vi "SwerveHeadingLock.vi"(1 "Max Driver Translation Joystick":dbl, 3 "Driver Rotation Joystick":dbl, 6 "PID Tuning Parameters":T1={"Kp"=0.1, "Ki"=0.1, "Kd"=0.1, "N-Diff"=10, "N-Int"=20, "Int Error Window"=0.5, "Max Ouput"=1.0, "Min Output"=-1.0, "Square Derivative"=FALSE, "N-Prop"=1} {"N-Prop" min=1; "Int Error Window" min=0.0; "N-Int" min=2; "N-Diff" min=2; "Kd" min=0.0; "Ki" min=0.0; "Kp" min=0.0}, 8 "Deceleration Hysteresis (ms)":u32, 10 "Heading Lock Strafe Deadband (ft/s)":dbl, 12 "External Disables":bool) -> (14 "Controller Summary":T2(graph), 17 "Joystick Rotation":dbl, 19 "Heading Lock":bool)   [LabVIEW 2020]
doc: "This VI runs a PID controller to maintain the robot's heading while translating above a specified velocity. Dropping below the velocity threshold or manually commanding a rotation will switch off the heading lock. Assumes that all of the joystick deadbands and scalings have already been applied."
uses:
  sensordata.vi
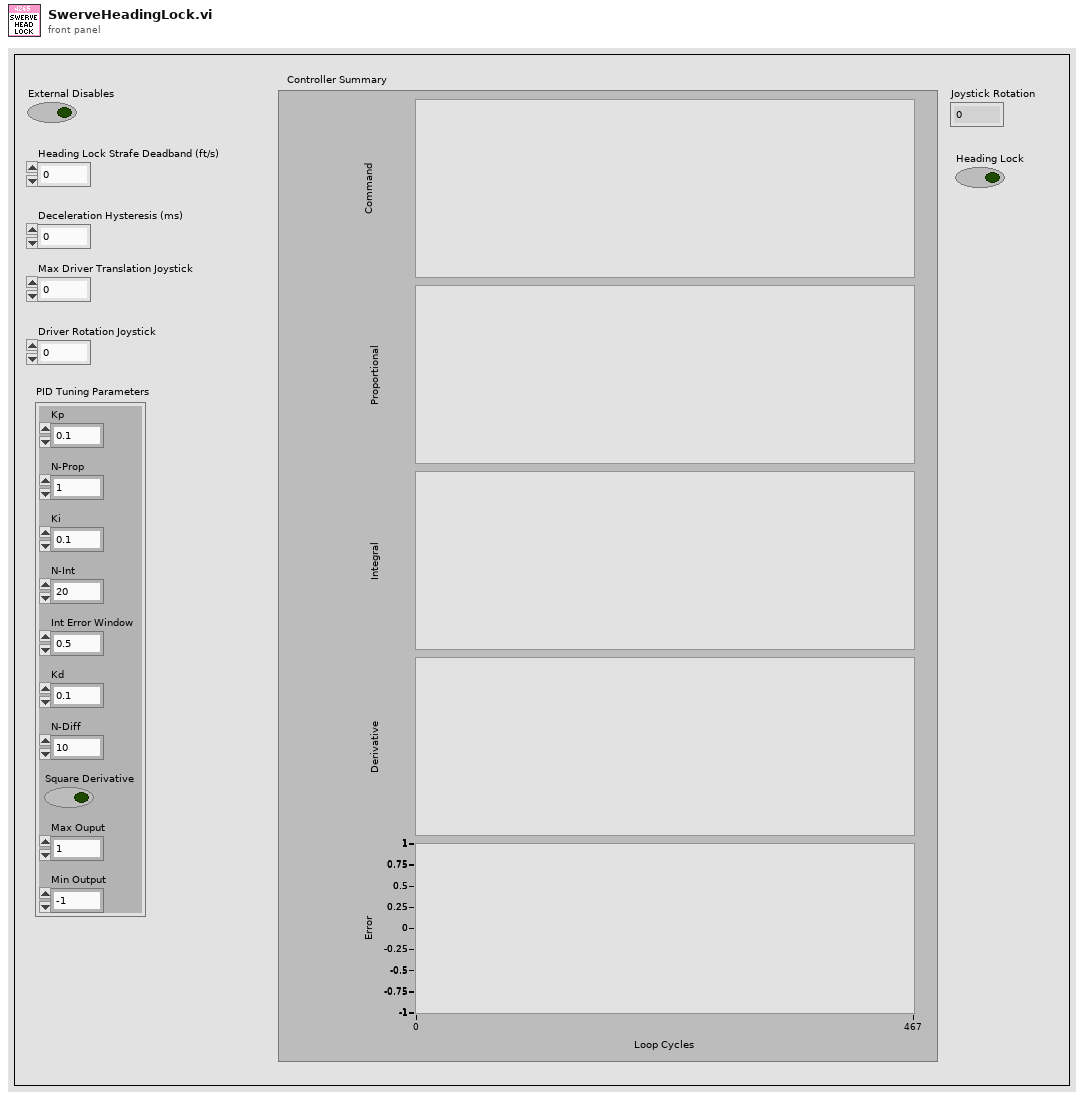
[diagram p1: front panel]
types:
  T1 = cluster{"Kp":dbl, "Ki":dbl, "Kd":dbl, "N-Diff":i32, "N-Int":i32, "Int Error Window":dbl, "Max Ouput":dbl, "Min Output":dbl, "Square Derivative":bool, "N-Prop":i32}
  T2 = cluster{"Command":dbl, "Proportional":dbl, "Integral":dbl, "Derivative":dbl, "Goal":dbl}
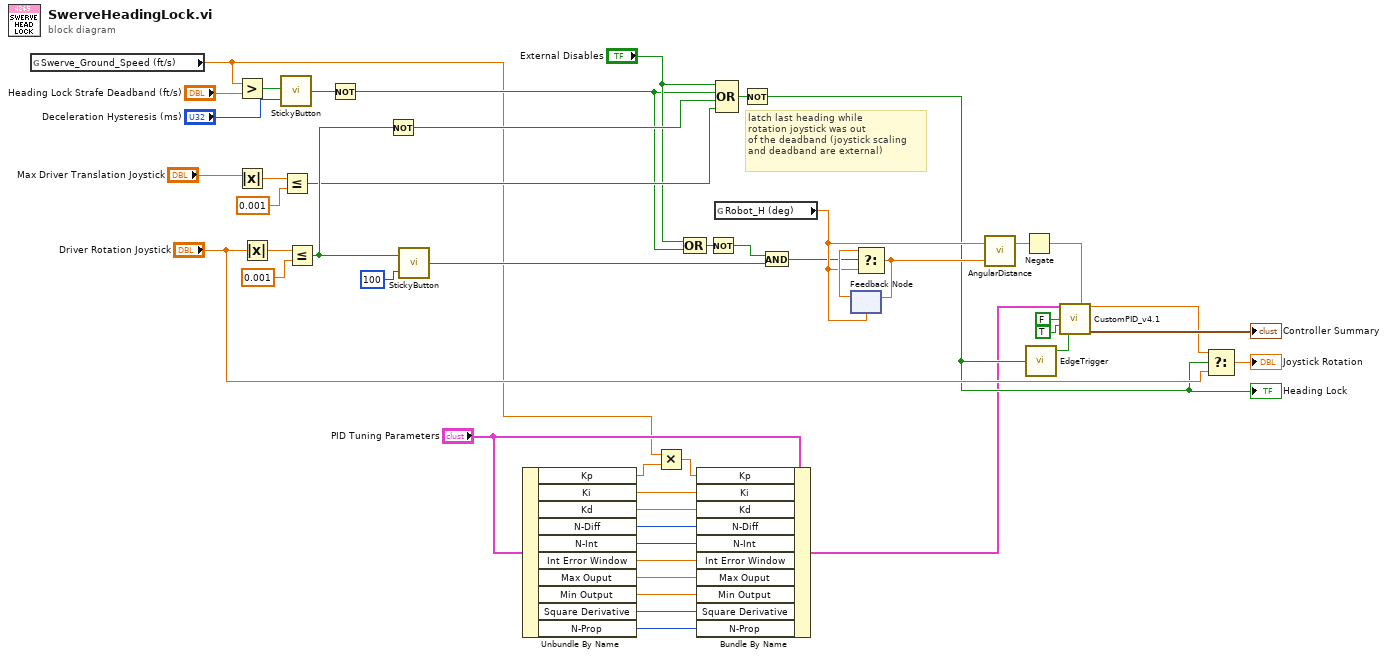
[diagram p0: block diagram]
diagram:
  # "latch last heading while\nrotation joystick was out \nof the deadband (joystick scaling \nand deadband are external)"
  n1 = global read "sensordata.vi" "Swerve_Ground_Speed (ft/s)"() -> (w5:dbl)
  n2 = Greater?(x=w5, y="Heading Lock Strafe Deadband (ft/s)") -> (0:w15:bool)
  n3 = Absolute Value(x="Max Driver Translation Joystick") -> (abs(x)=w13:dbl)
  n4 = Absolute Value(x="Driver Rotation Joystick") -> (abs(x)=w43:dbl)
  n5 = call "StickyButton.vi"("Time threshold (ms)"="Deceleration Hysteresis (ms)", "Button Input"=w15) -> ("Sticky Button"=w14:bool)
  n6 = Less Or Equal?(x=w13, y=0.001) -> (x <= y?=w10:bool)
  n7 = Less Or Equal?(x=w43, y=0.001) -> (x <= y?=w17:bool)
  n8 = Not(x=w14) -> (.not. x?=w8:bool)
  n9 = Not(x=w17) -> (.not. x?=w35:bool)
  n10 = call "StickyButton.vi"("Time threshold (ms)"=u32 100 ("y"), "Button Input"=w17) -> ("Sticky Button"=w31:bool)
  n11 = Unbundle By Name("PID Tuning Parameters") -> ("Kp"=w6:dbl, "Ki"=w1:dbl, "Kd"=w27:dbl, "N-Diff"=w26:i32, "N-Int"=w25:i32, "Int Error Window"=w24:dbl, "Max Ouput"=w23:dbl, "Min Output"=w22:dbl, "Square Derivative"=w21:bool, "N-Prop"=w20:i32)
  n12 = Multiply(x=w5, y=w6) -> (x*y=w4:dbl)
  n13 = Compound Arithmetic op=OR("External Disables", w8) -> (w7:bool)
  n14 = Bundle By Name(cluster="PID Tuning Parameters", "Kp"=w4, "Ki"=w1, "Kd"=w27, "N-Diff"=w26, "N-Int"=w25, "Int Error Window"=w24, "Max Ouput"=w23, "Min Output"=w22, "Square Derivative"=w21, "N-Prop"=w20) -> (w19:T1)
  n15 = Not(x=w7) -> (.not. x?=w30:bool)
  n16 = global read "sensordata.vi" "Robot_H (deg)"() -> (w36:dbl)
  n17 = Compound Arithmetic op=OR("External Disables", w8, w35, w10) -> (w34:bool)
  n18 = Not(x=w34) -> (.not. x?=w33:bool)
  "Heading Lock" <- w33
  n19 = And(x=w30, y=w31) -> (x .and. y?=w29:bool)
  n20 = feedback #1(w36) -> (w37:dbl)
  n21 = Select(t=w37, s=w29, f=w36) -> (s? t:f=w44:dbl)
  n22 = feedback-in #1(w44) -> ()
  n23 = call "AngularDistance.vi"("Goal Angle (deg) [0,360]"=w44, "Current Angle (deg) [-Inf,+Inf]"=w36) -> ("Signed Angular Distance (deg) [-180,+180]"=w3:dbl)  [unwired: 1 out]
  n24 = Negate(x=w3) -> (-x=w2:dbl)
  n25 = call "EdgeTrigger.vi"("Input Signal"=w33) -> ("Rising Edge Trigger"=w45:bool)  [unwired: 2 out]
  n26 = call "CustomPID_v4.1.vi"("PID Tuning Parameters"=w19, "Custom Error Calculation"=w2, "Reset on Goal Change ?"=FALSE, "Use Custom Error Calculation ?"=TRUE, "Reinit"=w45) -> ("Command"=w18:dbl, "Controller Summary"=→"Controller Summary":T2)  [unwired: 7 in, 2 out]
  n27 = Select(t=w18, s=w33, f="Driver Rotation Joystick") -> (s? t:f=→"Joystick Rotation":dbl)
